vi "StartStop Generation.vi"(8 "error in (no error)":errorcluster, 10 "Start/Stop":bool, 11 "Function Generator Actor in":refnum<class "Function Generator Actor.lvclass">) -> (0 "error out":errorcluster, 3 "Function Generator Actor out":refnum<class "Function Generator Actor.lvclass">)   [LabVIEW 2020, in "Function Generator Actor.lvlib" / "Function Generator Actor.lvclass"]
uses:
  Function Generator Actor.lvclass
  Function Generator Actor.lvclass/Function Generator Actor.ctl
  Signal Generation/Signal Generation Messages/StartStop Msg/StartStop Msg.lvclass/StartStop Msg.ctl
  <vilib>/ActorFramework/Message Enqueuer/Message Enqueuer.lvclass/Message Enqueuer.ctl
  <vilib>/ActorFramework/Message Enqueuer/Enqueue.vi
  Signal Generation/Signal Generation Messages/StartStop Msg/StartStop Msg.lvclass
  C:/Program Files (x86)/National Instruments/LabVIEW 2020/vi.lib/ActorFramework/Message/Message.lvclass
  <vilib>/ActorFramework/Message Priority Queue/Priority Enqueue.vi
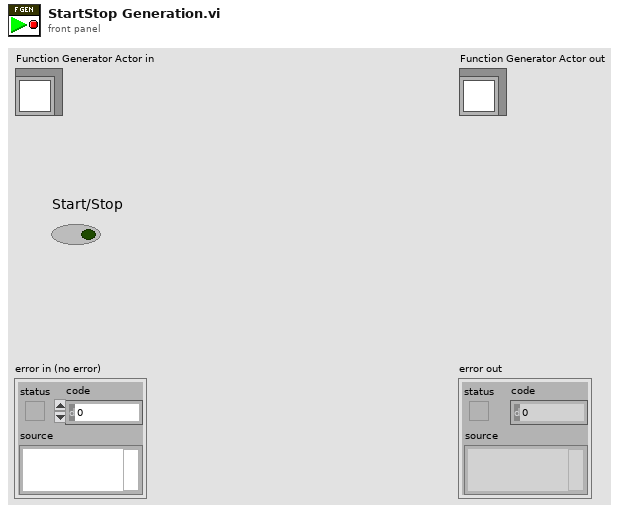
[diagram p1: front panel]
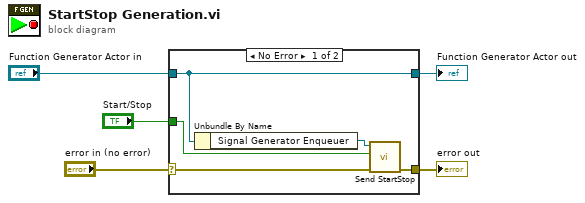
[diagram p0: block diagram]
diagram:
  n1 = case shown="No Error" "error in (no error)" {
    selector: "error in (no error)" -> [w8 w12]
    tunnel: [w7 w12] -> w4
    tunnel: [w10 w11] -> w2
    tunnel: "Function Generator Actor in" -> [w10 w11]
    tunnel: "Start/Stop" -> [w6 _]
    frame No Error {
      n2 = Unbundle By Name(w10) -> ("Signal Generator Enqueuer"=w9:refnum<class "Message Enqueuer.lvclass">)
      n3 = call "Send StartStop.vi"("error in (no error)"=w8, "Start/Stop"=w6, "Message Enqueuer"=w9) -> ("error out"=w7:errorcluster)  [unwired: 7 in, 1 out]
    }
    frame Error {
    }
  }
  "error out" <- w4
  "Function Generator Actor out" <- w2
